vi "OSC_Red_Calc.vi"(7 "Ox Calc Flow":dbl, 8 "Flow":dbl, 9 "Lambda 2 Array":dbl[](array[numeric]), 10 "Lambda 1 Array":dbl[](array[numeric]), 11 "MFC":dbl) -> (0 "OSC MFC":dbl, 1 "OSC-Meas Flow":dbl, 2 "OSC- Calc Flow":dbl, 3 "Calculated Flow":dbl, 4 "Time":dbl)   [LabVIEW 2014]
uses:
  <vilib>/Analysis/baseanly.llb/Mean (DBL).vi
  <vilib>/Analysis/NI_AALPro.lvlib
  <vilib>/Analysis/NI_AALBase.lvlib
panel:
  out "L1 TP 2":i32
  out "Value 2":dbl
  out "L2 TP 2":i32
  out "Value":dbl
  out "mean":dbl format="%0.2f"
  out "mean 2":dbl format="%0.2f"
  out "mean 3":dbl format="%0.2f"
  out "L1 Gradient":dbl[](graph)
  out "L1 Data":dbl[](graph)
  out "L1 Max Grad":dbl
  out "L1 TP":i32
  out "L2 Gradient":dbl[](graph)
  out "L2 Data":dbl[](graph)
  out "L2 Max Grad":dbl
  out "L2 TP":i32
  # "OSC Calculation"
  # "Inputs"
  # "Outputs"
  # "Indicators"
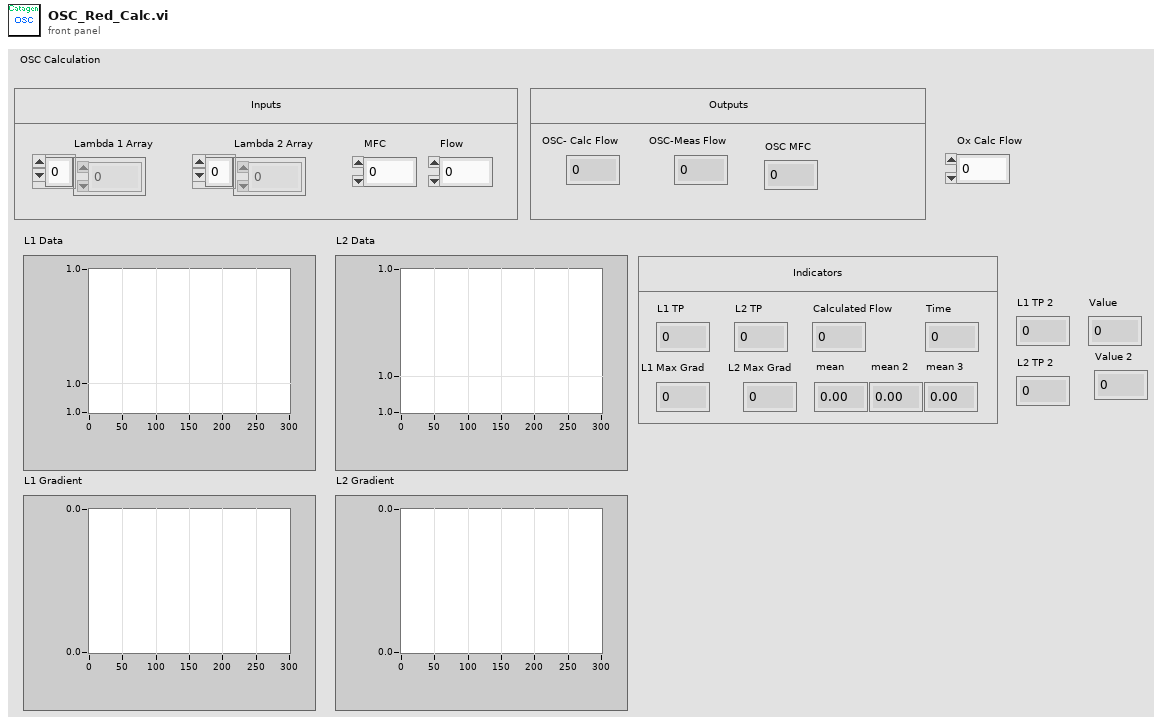
[diagram p1: front panel]
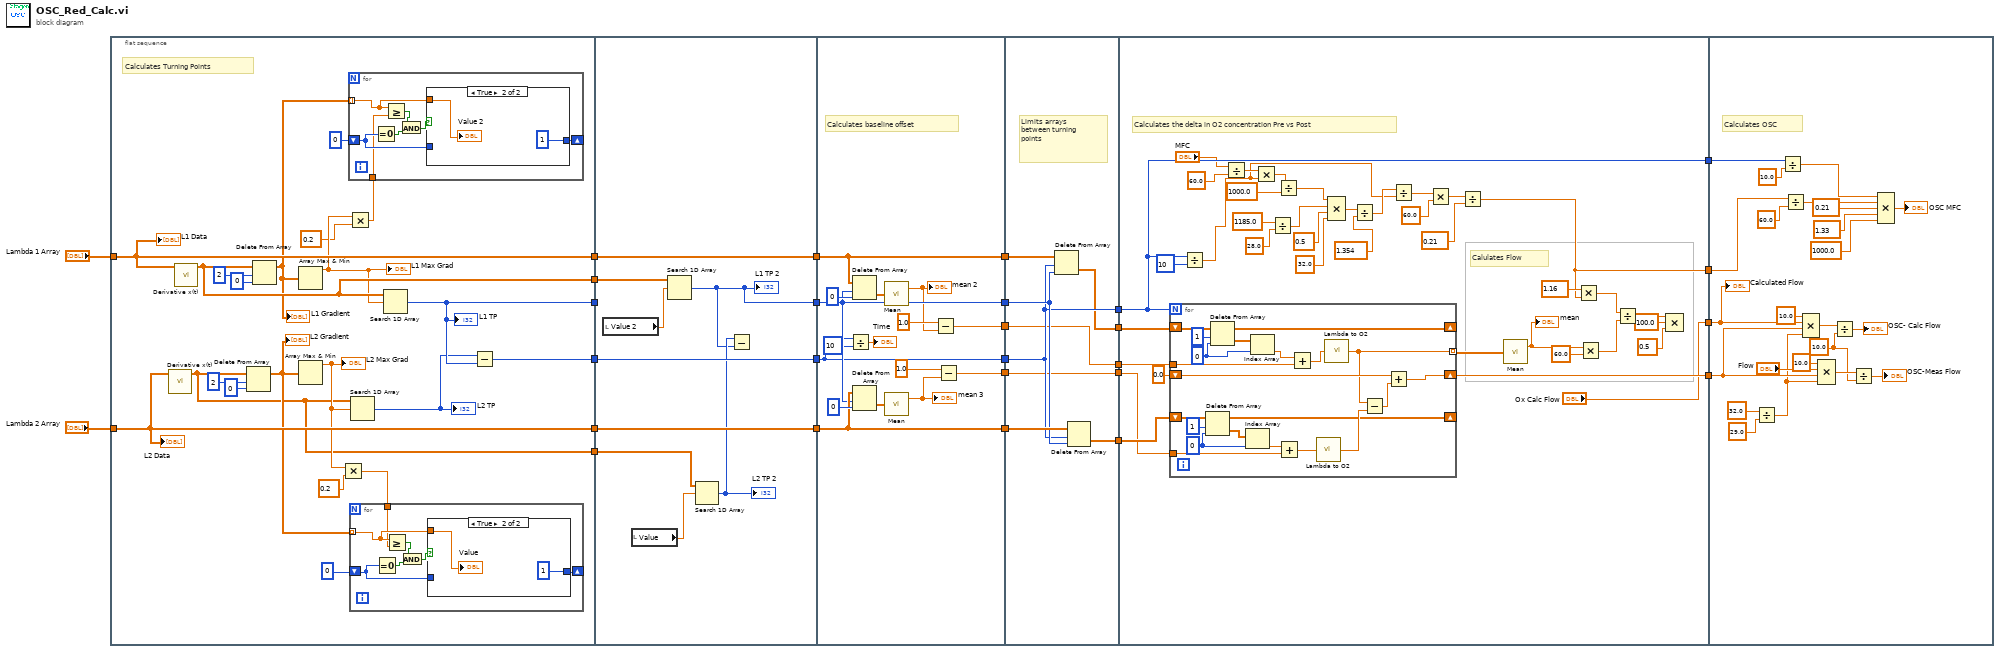
[diagram p0: block diagram]
diagram:
  n1 = flat-sequence {
    tunnel: [w40] -> w10
    tunnel: [w41] -> w8
    tunnel: [w44] -> w6
    tunnel: [w43] -> w4
    tunnel: "Lambda 1 Array" -> [w41]
    tunnel: "Lambda 2 Array" -> [w40]
    tunnel: [w34] -> w2
    tunnel: [w33] -> w1
    tunnel: w10 -> [w77]
    tunnel: [w77] -> w9
    tunnel: w8 -> [w76]
    tunnel: [w76] -> w7
    tunnel: w6 -> [w75]
    tunnel: [w75] -> w5
    tunnel: w4 -> [_]
    tunnel: [w69] -> w3
    tunnel: w2 -> [w73]
    tunnel: w1 -> [w72]
    tunnel: w9 -> [w88]
    tunnel: [w88] -> w27
    tunnel: w7 -> [w93]
    tunnel: [w93] -> w26
    tunnel: w5 -> [w80]
    tunnel: [w80] -> w25
    tunnel: w3 -> [w87]
    tunnel: [w87] -> w24
    tunnel: [w85] -> w23
    tunnel: [w81] -> w14
    tunnel: w27 -> [w100]
    tunnel: w26 -> [w101]
    tunnel: w25 -> [w98]
    tunnel: w24 -> [w99]
    tunnel: [w98] -> w22
    tunnel: [w97] -> w21
    tunnel: [w96] -> w20
    tunnel: w23 -> [w95]
    tunnel: [w95] -> w19
    tunnel: w14 -> [w94]
    tunnel: [w94] -> w13
    tunnel: w22 -> [w111]
    tunnel: w21 -> [w138]
    tunnel: w20 -> [w139]
    tunnel: [w136] -> w18
    tunnel: ["Ox Calc Flow"] -> w17
    tunnel: w19 -> [w126]
    tunnel: w13 -> [w125]
    tunnel: [w111] -> w12
    tunnel: [w108] -> w11
    tunnel: w18 -> [w178]
    tunnel: w17 -> [w182]
    tunnel: w12 -> [w162]
    tunnel: w11 -> [w161]
    frame #0 {
      # "Calculates Turning Points"
      n2 = call <vilib>:"Derivative x(t).vi"("X"=w40) -> ("dX/dt"=w34:dbl[])  [unwired: 9 in, 1 out]
      n3 = call <vilib>:"Derivative x(t).vi"("X"=w41) -> ("dX/dt"=w33:dbl[])  [unwired: 9 in, 1 out]
      n4 = Delete From Array(array=w34, length=2, index=0) -> (array with subset deleted=w38:dbl[])  [unwired: 1 out]
      "L2 Gradient" <- w38
      n5 = Delete From Array(array=w33, length=2, index=0) -> (array with subset deleted=w32:dbl[])  [unwired: 1 out]
      "L1 Gradient" <- w32
      n6 = Array Max & Min(array=w32) -> (max value=w30:dbl)  [unwired: 3 out]
      "L1 Max Grad" <- w30
      n7 = Array Max & Min(array=w38) -> (max value=w35:dbl)  [unwired: 3 out]
      "L2 Max Grad" <- w35
      n8 = Multiply(x=w35, y=0.2) -> (x*y=w37:dbl)
      n9 = Multiply(x=w30, y=0.2) -> (x*y=w31:dbl)
      n10 = for {
        tunnel: w32 -> [w51] mode=indexing
        shift-right: [w53] -> _
        shift-left: 0 ("index") -> [w50]
        tunnel: w31 -> [w49]
        n11 = Equal To 0?(x=w50) -> (x = 0?=w52:bool)
        n12 = Greater Or Equal?(x=w51, y=w49) -> (x >= y?=w54:bool)
        n13 = And(x=w54, y=w52) -> (x .and. y?=w55:bool)
        n14 = case shown="True" w55 {
          tunnel: [w56 1 ("index")] -> w53
          tunnel: w51 -> [_ w57]
          tunnel: w50 -> [w56 _]
          frame False {
          }
          frame True {
            "Value 2" <- w57
          }
        }
      }
      n15 = for {
        tunnel: w38 -> [w61] mode=indexing
        shift-right: [w63] -> _
        shift-left: 0 ("index") -> [w60]
        tunnel: w37 -> [w59]
        n16 = Equal To 0?(x=w60) -> (x = 0?=w62:bool)
        n17 = Greater Or Equal?(x=w61, y=w59) -> (x >= y?=w64:bool)
        n18 = And(x=w64, y=w62) -> (x .and. y?=w65:bool)
        n19 = case shown="True" w65 {
          tunnel: [w66 1 ("index")] -> w63
          tunnel: w61 -> [_ w67]
          tunnel: w60 -> [w66 _]
          frame False {
          }
          frame True {
            "Value" <- w67
          }
        }
      }
      n20 = Search 1D Array(1D array=w34, element=w35) -> (index of element=w42:i32)  [unwired: 1 in]
      "L2 TP" <- w42
      n21 = Search 1D Array(1D array=w33, element=w30) -> (index of element=w43:i32)  [unwired: 1 in]
      "L1 TP" <- w43
      n22 = Subtract(x=w42, y=w43) -> (x-y=w44:i32)
      "L1 Data" <- w41
      "L2 Data" <- w40
    }
    frame #1 {
      n23 = local read "Value 2"() -> (w71:dbl)
      n24 = local read "Value"() -> (w74:dbl)
      n25 = Search 1D Array(1D array=w72, element=w71) -> (index of element=w69:i32)  [unwired: 1 in]
      "L1 TP 2" <- w69
      n26 = Search 1D Array(1D array=w73, element=w74) -> (index of element=w70:i32)  [unwired: 1 in]
      "L2 TP 2" <- w70
      n27 = Subtract(x=w70, y=w69) -> ()  [unwired: 1 out]
    }
    frame #2 {
      # "Calculates baseline offset"
      n28 = Divide(x=w80, y=10) -> (x/y=→"Time":dbl)
      n29 = Delete From Array(array=w93, length=w87, index=0) -> (deleted portion=w91:dbl[])  [unwired: 1 out]
      n30 = Delete From Array(array=w88, length=w87, index=0) -> (deleted portion=w90:dbl[])  [unwired: 1 out]
      n31 = call-poly <vilib>:"Mean.vi"("X"=w91) -> ("mean"=w83:dbl)  [unwired: 1 out]
      "mean 2" <- w83
      n32 = call-poly <vilib>:"Mean.vi"("X"=w90) -> ("mean"=w86:dbl)  [unwired: 1 out]
      "mean 3" <- w86
      n33 = Subtract(x=1.0, y=w83) -> (x-y=w81:dbl)
      n34 = Subtract(x=1.0, y=w86) -> (x-y=w85:dbl)
    }
    frame #3 {
      # "Limits arrays\nbetween turning\npoints"
      n35 = Delete From Array(array=w101, length=w98, index=w99) -> (deleted portion=w96:dbl[])  [unwired: 1 out]
      n36 = Delete From Array(array=w100, length=w98, index=w99) -> (deleted portion=w97:dbl[])  [unwired: 1 out]
    }
    frame #4 {
      # "Calculates the delta in O2 concentration Pre vs Post"
      # "Calulates Flow"
      n37 = for {
        N: w111 -> [_]
        shift-right: [w147] -> _
        shift-left: w139 -> [w160]
        shift-right: [w146] -> _
        shift-left: w138 -> [w153]
        shift-right: [w151] -> w136
        shift-left: 0.0 ("element") -> [w152]
        tunnel: [w148] -> w135 mode=indexing
        tunnel: w126 -> [w144]
        tunnel: w125 -> [w141]
        w156 = 0 ("index")
        w157 = 0 ("index")
        n38 = Delete From Array(array=w153, length=1, index=w156) -> (deleted portion=w155:dbl[], array with subset deleted=w146:dbl[])
        n39 = Delete From Array(array=w160, length=1, index=w157) -> (deleted portion=w158:dbl[], array with subset deleted=w147:dbl[])
        n40 = Index Array(array=w155, index=w156) -> (element=w145:dbl)
        n41 = Index Array(array=w158, index=w157) -> (element=w142:dbl)
        n42 = Add(x=w145, y=w144) -> (x+y=w143:dbl)
        n43 = Add(x=w142, y=w141) -> (x+y=w140:dbl)
        n44 = call "Lambda to O2.vi"("Lambda"=w143) -> ("O2 %"=w149:sgl)
        n45 = call "Lambda to O2.vi"("Lambda"=w140) -> ("O2 %"=w148:sgl)
        n46 = Subtract(x=w148, y=w149) -> (x-y=w150:sgl)
        n47 = Add(x=w152, y=w150) -> (x+y=w151:dbl)
      }
      n48 = Divide(x=w111, y=10) -> (x/y=w110:dbl)
      n49 = Divide(x="MFC", y=60.0) -> (x/y=w114:dbl)
      n50 = Multiply(x=w114, y=w110) -> (x*y=w106:dbl)
      n51 = Divide(x=1185.0, y=28.0) -> (x/y=w115:dbl)
      n52 = Divide(x=w106, y=1000.0) -> (x/y=w105:dbl)
      n53 = Compound Arithmetic op=MULTIPLY(w105, w115, 0.5 ("y"), 32.0 ("y")) -> (w118:dbl)
      n54 = Divide(x=w118, y=1.354 ("x")) -> (x/y=w120:dbl)
      n55 = Divide(x=w120, y=w110) -> (x/y=w121:dbl)
      n56 = Multiply(x=w121, y=60.0) -> (x*y=w123:dbl)
      n57 = Divide(x=w123, y=0.21) -> (x/y=w108:dbl)
      n58 = call-poly <vilib>:"Mean.vi"("X"=w135) -> ("mean"=w133:dbl)  [unwired: 1 out]
      "mean" <- w133
      n59 = Multiply(x=1.16, y=w108) -> (x*y=w131:dbl)
      n60 = Multiply(x=w133, y=60.0) -> (x*y=w130:dbl)
      n61 = Divide(x=w131, y=w130) -> (x/y=w129:dbl)
      n62 = Compound Arithmetic op=MULTIPLY(w129, 100.0 ("value"), 0.5 ("value")) -> ()  [unwired: 1 out]
    }
    frame #5 {
      w171 = 10.0 ("y")
      # "Calculates OSC"
      n63 = Divide(x=32.0, y=29.0) -> (x/y=w176:dbl)
      n64 = Divide(x=w162, y=10.0) -> (x/y=w164:dbl)
      n65 = Divide(x=w161, y=60.0) -> (x/y=w169:dbl)
      n66 = Compound Arithmetic op=MULTIPLY(10.0 ("value"), w182, w178, w176) -> (w172:dbl)
      n67 = Compound Arithmetic op=MULTIPLY(10.0 ("value"), "Flow", w178, w176) -> (w173:dbl)
      n68 = Divide(x=w172, y=w171) -> (x/y=→"OSC- Calc Flow":dbl)
      n69 = Divide(x=w173, y=w171) -> (x/y=→"OSC-Meas Flow":dbl)
      n70 = Compound Arithmetic op=MULTIPLY(w164, w169, 0.21 ("value"), 1.33 ("value"), 1000.0 ("value")) -> (→"OSC MFC":dbl)
      "Calculated Flow" <- w182
    }
  }
